vi "createState.vi"(8 "error in (no error)":errorcluster, 10 "State:":T1=enum."EndingCycleState", 11 "StateFactory in":refnum<class "StateFactory.lvclass">) -> (0 "error out":errorcluster, 2 "State.lvclass":refnum<class "State.lvclass">, 3 "StateFactory out":refnum<class "StateFactory.lvclass">)   [LabVIEW 2013, in "StateFactory.lvclass"]
uses:
  StateFactory.lvclass
  Typedefs/StateSelector.ctl
  State/State.lvclass
  States/AwaitingSetpointAcknowledgmentState/AwaitingSetpointAcknowledgmentState.lvclass
  States/EndingCycleState/EndingCycleState.lvclass
  States/FaultState/FaultState.lvclass
  States/OffState/OffState.lvclass
  States/PausingState/PausingState.lvclass
  States/RequestingNewSetpointState/RequestingNewSetpointState.lvclass
  States/SamplingState/SamplingState.lvclass
  States/SettlingState/SettlingState.lvclass
  States/SoakingState/SoakingState.lvclass
  States/StabilizingState/StabilizingState.lvclass
  States/StandbyState/StandbyState.lvclass
  States/StoppedState/StoppedState.lvclass
  States/TransitioningTemperatureState/TransitioningTemperatureState.lvclass
  Typedefs/AITDTTypedefs.lvlib
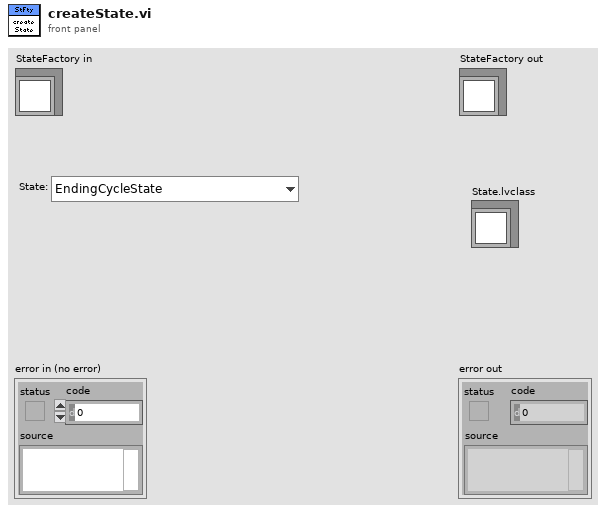
[diagram p1: front panel]
types:
  T1 = typedef "AITDTTypedefs.lvlib/StateSelector.ctl" = enum16{"AwaitingSetpointAcknowledgmentState", "EndingCycleState", "FaultState", "OffState", "PausingState", "RequestingNewSetpointState", "SamplingState", "SettlingState", "SoakingState", "StabilizingState", "StandbyState", "StoppedState", "TransitioningTemperatureState"}
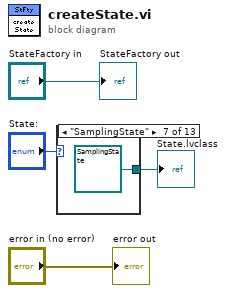
[diagram p0: block diagram]
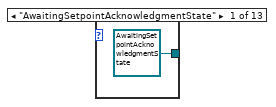
[diagram p2: hidden frame]
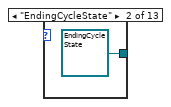
[diagram p3: hidden frame]
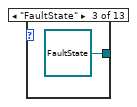
[diagram p4: hidden frame]
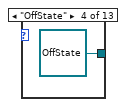
[diagram p5: hidden frame]
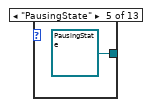
[diagram p6: hidden frame]
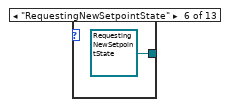
[diagram p7: hidden frame]
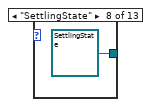
[diagram p8: hidden frame]
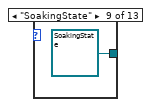
[diagram p9: hidden frame]
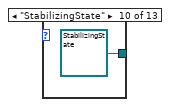
[diagram p10: hidden frame]
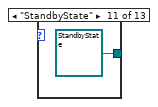
[diagram p11: hidden frame]
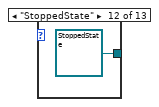
[diagram p12: hidden frame]
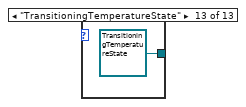
[diagram p13: hidden frame]
diagram:
  n1 = case shown="\"SamplingState\"" "State:" {
    tunnel: [refnum<class "AwaitingSetpointAcknowledgmentState.lvclass"> refnum ("AwaitingSetpointAcknowledgmentState.lvclass") refnum<class "EndingCycleState.lvclass"> refnum ("EndingCycleState.lvclass") refnum<class "FaultState.lvclass"> refnum ("FaultState.lvclass") refnum<class "OffState.lvclass"> refnum ("ShutdownState.lvclass") refnum<class "PausingState.lvclass"> refnum ("PausingState.lvclass") refnum<class "RequestingNewSetpointState.lvclass"> refnum ("RequestingNewSetpointState.lvclass") refnum<class "SamplingState.lvclass"> refnum ("SamplingState.lvclass") refnum<class "SettlingState.lvclass"> refnum ("SettlingState.lvclass") refnum<class "SoakingState.lvclass"> refnum ("SoakingState.lvclass") refnum<class "StabilizingState.lvclass"> refnum ("StabilizingState.lvclass") refnum<class "StandbyState.lvclass"> refnum ("StandbyState.lvclass") refnum<class "StoppedState.lvclass"> refnum ("StoppedState.lvclass") refnum<class "TransitioningTemperatureState.lvclass"> refnum ("TransitioningTemperatureState.lvclass")] -> w1
    frame "AwaitingSetpointAcknowledgmentState" {
    }
    frame "EndingCycleState" {
    }
    frame "FaultState" {
    }
    frame "OffState" {
    }
    frame "PausingState" {
    }
    frame "RequestingNewSetpointState" {
    }
    frame "SamplingState" {
    }
    frame "SettlingState" {
    }
    frame "SoakingState" {
    }
    frame "StabilizingState" {
    }
    frame "StandbyState" {
    }
    frame "StoppedState" {
    }
    frame "TransitioningTemperatureState" {
    }
  }
  "State.lvclass" <- w1
  "error out" <- "error in (no error)"
  "StateFactory out" <- "StateFactory in"
